vi "ziOpen.vi"(3 "Error In":errorcluster, 4 "Port obsolete (auto)":u16, 5 "Hostname obsolete (auto)":string, 6 "Address":string="DEV") -> (0 "Error Out":errorcluster, 1 "Selected Device":string, 2 "HandleOut":T1 {"Handle" format="0x%08x"; "Conn" format="0x%08x"})   [LabVIEW 2009, in "Zurich Instruments LabOne.lvlib"]
doc: "Creates a connection to a Data Server. <b>Address</b> is of the format {<host>}{:<port}{::<Device ID>}. Usually it is sufficient to provide the <b>Device ID</b> only. The host and port are then determined by network discovery. Should the discovery not work, prepend <host>:<port>:: to the Device ID. Examples are \"myhf2.company.com:8004::dev466\" or \"myhf2.company.com:8004\". In the latter case the first found instrument on the data server listening on myhf2.company.com:8004 will be selected."
uses:
  <instrlib>/Zurich Instruments LabOne/Zurich Instruments LabOne.lvlib
  <instrlib>/Zurich Instruments LabOne/Public/ziTypeHandle.ctl
  <instrlib>/Zurich Instruments LabOne/Public/ziTypeDisovery.ctl
  <instrlib>/Zurich Instruments LabOne/Private/ziLV64.dll
panel:
  out "auto-connected":bool
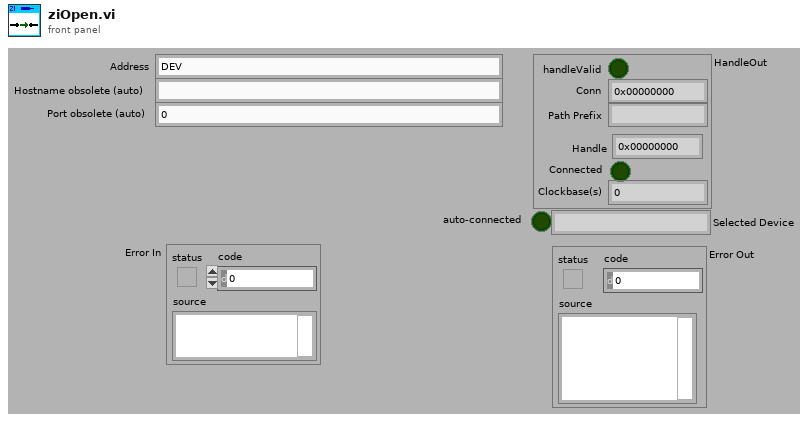
[diagram p1: front panel]
types:
  T1 = typedef "Zurich Instruments LabOne.lvlib/ziTypeHandle.ctl" = cluster{"handleValid":bool, "Conn":u64, "Path Prefix":string, "Handle":u64, "Connected":bool, "Clockbase(s)":dbl}
  T2 = typedef "Zurich Instruments LabOne.lvlib/ziTypeDisovery.ctl" = cluster{"timestamp":u64, "deviceid":string, "devicetype":string, "serveraddress":string, "serverport":u32, "apilevel":u32, "discoverable":bool, "interface":string, "connected":string, "available":bool, "owner":string, "status":string, "options ":string, "serverversion":string}
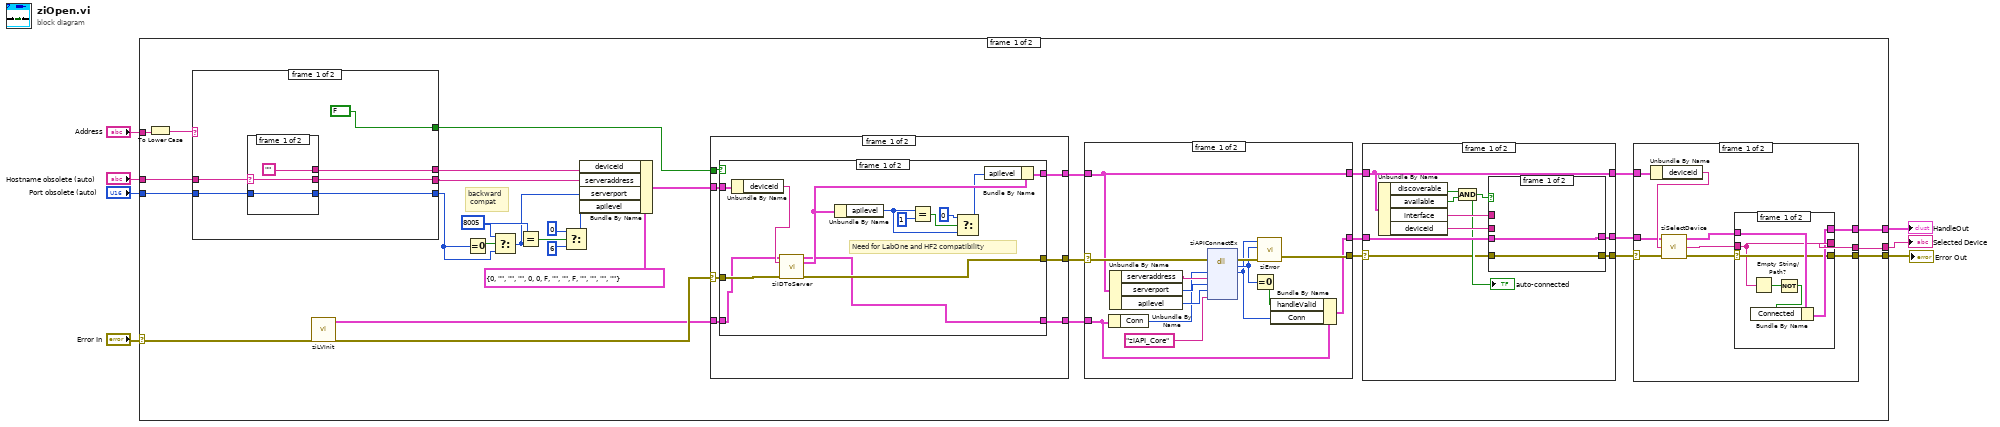
[diagram p0: block diagram]
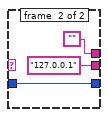
[diagram p2: hidden frame]
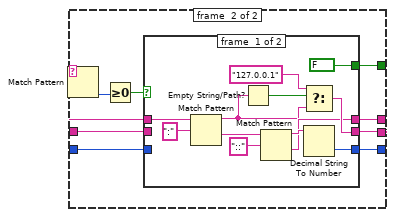
[diagram p3: hidden frame]
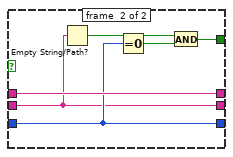
[diagram p4: hidden frame]
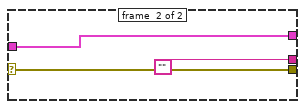
[diagram p6: hidden frame]
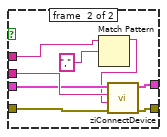
[diagram p7: hidden frame]
diagram:
  n1 = case shown="No Error" "Error In" {
    selector: "Error In" -> [w12 w168]
    tunnel: [w39 w168] -> w7
    tunnel: [w38 _] -> w6
    tunnel: "Hostname obsolete (auto)" -> [w31 _]
    tunnel: "Port obsolete (auto)" -> [w32 _]
    tunnel: [w37 _] -> w5
    tunnel: "Address" -> [w9 _]
    frame #0 {
      w18 = u32 8005
      # "backward\n compat"
      n2 = To Lower Case(string=w9) -> (all lower case string=w8:string)
      n3 = case shown="\"\", \"dev\"" w8 {
        selector: w8 -> [_ w54]
        tunnel: w31 -> [w45 w60]
        tunnel: w32 -> [w44 w56]
        tunnel: [w43 w61] -> w19
        tunnel: [w42 w59] -> w25
        tunnel: [w41 w58] -> w24
        tunnel: [FALSE w57] -> w21
        frame #0 {
          n4 = case shown="\"\"" w45 {
            selector: w45 -> [w47 _]
            tunnel: w44 -> [w46 w51]
            tunnel: [w46 w51] -> w43
            tunnel: [w47 "127.0.0.1"] -> w42
            tunnel: ["" ""] -> w41
            frame #0 {
            }
            frame #1 {
            }
          }
        }
        frame #1 {
          n5 = Match Pattern(string=w54, regular expression=":") -> (offset past match=w55:i32)  [unwired: 1 in, 3 out]
          n6 = Greater Or Equal To 0?(x=w55) -> (x >= 0?=w52:bool)
          n7 = case shown="False" w52 {
            tunnel: [w66 w78] -> w61
            tunnel: w60 -> [_ w75]
            tunnel: [w68 w75] -> w59
            tunnel: w54 -> [w72 w79]
            tunnel: [w65 w79] -> w58
            tunnel: [FALSE w76] -> w57
            tunnel: w56 -> [_ w78]
            frame #0 {
              n8 = Match Pattern(string=w72, regular expression=":") -> (before substring=w63:string, after substring=w69:string)  [unwired: 1 in, 2 out]
              n9 = Empty String/Path?(string/path=w63) -> (empty?=w62:bool)
              n10 = Match Pattern(string=w69, regular expression="::") -> (before substring=w67:string, after substring=w65:string)  [unwired: 1 in, 2 out]
              n11 = Select(t="127.0.0.1", s=w62, f=w63) -> (s? t:f=w68:string)
              n12 = Decimal String To Number(string=w67) -> (number=w66:i32)  [unwired: 2 in, 1 out]
            }
            frame #1 {
              n13 = Empty String/Path?(string/path=w75) -> (empty?=w74:bool)
              n14 = Equal To 0?(x=w78) -> (x = 0?=w77:bool)
              n15 = And(x=w74, y=w77) -> (x .and. y?=w76:bool)
            }
          }
        }
      }
      n16 = call <instrlib>:"ziLVInit.vi"("Error In"=w12) -> ("Error Out"=w11:errorcluster, "ziHandle"=w10:T1)  [unwired: 9 in]
      n17 = Equal To 0?(x=w19) -> (x = 0?=w20:bool)
      n18 = Select(t=w18, s=w20, f=w19) -> (s? t:f=w13:u32)
      n19 = Equal?(x=w18, y=w13) -> (x = y?=w17:bool)
      n20 = Select(t=u32 0, s=w17, f=u32 6) -> (s? t:f=w14:u32)
      n21 = Bundle By Name(cluster=T2 {"timestamp"=0, "deviceid"="", "devicetype"="", "serveraddress"="", "serverport"=0, "apilevel"=0, "discoverable"=FALSE, "interface"="", "connected"="", "available"=FALSE, "owner"="", "status"="", "options "="", "serverversion"=""} ("ziDiscovery"), "deviceid"=w24, "serveraddress"=w25, "serverport"=w13, "apilevel"=w14) -> (w27:T2)
      n22 = case shown="No Error" w11 {
        selector: w11 -> [w131 w150]
        tunnel: [w130 w150] -> w33
        tunnel: [w129 w148] -> w30
        tunnel: w21 -> [w128 _]
        tunnel: w27 -> [w127 w148]
        tunnel: w10 -> [w126 w149]
        tunnel: [w125 w149] -> w23
        frame #0 {
          n23 = case shown="True" w128 {
            tunnel: w131 -> [w144 w147]
            tunnel: [w143 w147] -> w130
            tunnel: [w141 w146] -> w129
            tunnel: w127 -> [w135 w146]
            tunnel: w126 -> [w132 w145]
            tunnel: [w133 w145] -> w125
            frame #0 {
              # "Need for LabOne and HF2 compatibility"
              n24 = Unbundle By Name(w135) -> ("deviceid"=w134:string)
              n25 = call <instrlib>:"ziIDToServer.vi"("ziHandle In"=w132, "Device ID"=w134, "Error In"=w144) -> ("ziHandle Out"=w133:T1, "ziDiscovery"=w142:T2, "Error Out"=w143:errorcluster)  [unwired: 10 in]
              n26 = Unbundle By Name(w142) -> ("apilevel"=w137:u32)
              n27 = Equal?(x=w137, y=u32 1) -> (x = y?=w139:bool)
              n28 = Select(t=u32 0, s=w139, f=w137) -> (s? t:f=w136:u32)
              n29 = Bundle By Name(cluster=w142, "apilevel"=w136) -> (w141:T2)
            }
            frame #1 {
            }
          }
        }
        frame #1 {
        }
      }
      n30 = case shown="No Error" w33 {
        selector: w33 -> [w160 w167]
        tunnel: [w163 w167] -> w34
        tunnel: w30 -> [w157 w166]
        tunnel: [w157 w166] -> w29
        tunnel: w23 -> [w153 w165]
        tunnel: [w152 w165] -> w22
        frame #0 {
          n31 = Unbundle By Name(w153) -> ("Conn"=w155:u64)
          n32 = Unbundle By Name(w157) -> ("serveraddress"=w159:string, "serverport"=w158:u32, "apilevel"=w156:u32)
          n33 = dll-call lib="C:/Program Files/National Instruments/LabVIEW 2009/instr.lib/Zurich Instruments LabOne/Private/ziLV*.*" fn="ziAPIConnectEx"(error in=w160, "Conn"=w155, "hostname"=w159, "Port"=w158, "ZIAPIVersion_enum"=w156, "Implementation"="ziAPI_Core") -> (error out=w164:errorcluster, "return type"=w162:u32, "Conn"=w154:u64)  [unwired: 6 in, 1 out]
          n34 = Equal To 0?(x=w162) -> (x = 0?=w151:bool)
          n35 = call <instrlib>:"ziError.vi"("Conn"=w154, "ziErrorCode"=w162, "Error In"=w164) -> ("Error Out"=w163:errorcluster)  [unwired: 3 in]
          n36 = Bundle By Name(cluster=w153, "handleValid"=w151, "Conn"=w154) -> (w152:T1)
        }
        frame #1 {
        }
      }
      n37 = case shown="No Error" w34 {
        selector: w34 -> [w102 w123]
        tunnel: w29 -> [w103 w122]
        tunnel: w22 -> [w110 w124]
        tunnel: [w109 w124] -> w36
        tunnel: [w108 w123] -> w35
        tunnel: [w103 w122] -> w28
        frame #0 {
          n38 = Unbundle By Name(w103) -> ("discoverable"=w105:bool, "available"=w106:bool, "interface"=w107:string, "deviceid"=w111:string)
          n39 = And(x=w105, y=w106) -> (x .and. y?=w104:bool)
          "auto-connected" <- w104
          n40 = case shown="True" w104 {
            tunnel: w111 -> [_ w121]
            tunnel: w110 -> [w112 w117]
            tunnel: [w112 w120] -> w109
            tunnel: [w113 w119] -> w108
            tunnel: w107 -> [_ w114]
            tunnel: w102 -> [w113 w118]
            frame #0 {
            }
            frame #1 {
              n41 = Match Pattern(string=w114, regular expression="," ("replace string (\"\")")) -> (before substring=w116:string)  [unwired: 1 in, 3 out]
              n42 = call <instrlib>:"ziConnectDevice.vi"("Error In"=w118, "Device Interface"=w116, "Device Serial"=w121, "Handle In"=w117) -> ("Error Out"=w119:errorcluster, "Handle Out"=w120:T1)  [unwired: 6 in]
            }
          }
        }
        frame #1 {
        }
      }
      n43 = case shown="No Error" w35 {
        selector: w35 -> [w89 w99]
        tunnel: [w80 w99] -> w39
        tunnel: w36 -> [w86 w101]
        tunnel: [w83 w101] -> w38
        tunnel: [w81 ""] -> w37
        tunnel: w28 -> [w88 _]
        frame #0 {
          n44 = Unbundle By Name(w88) -> ("deviceid"=w87:string)
          n45 = call <instrlib>:"ziSelectDevice.vi"("Error In"=w89, "Device (first)"=w87, "Handle In"=w86) -> ("Error Out"=w85:errorcluster, "Selected Device"=w82:string, "Handle Out"=w84:T1)
          n46 = case shown="No Error" w85 {
            selector: w85 -> [w93 w96]
            tunnel: w84 -> [w95 w98]
            tunnel: w82 -> [w92 w97]
            tunnel: [w94 w98] -> w83
            tunnel: [w92 w97] -> w81
            tunnel: [w93 w96] -> w80
            frame #0 {
              n47 = Empty String/Path?(string/path=w92) -> (empty?=w91:bool)
              n48 = Not(x=w91) -> (.not. x?=w90:bool)
              n49 = Bundle By Name(cluster=w95, "Connected"=w90) -> (w94:T1)
            }
            frame #1 {
            }
          }
        }
        frame #1 {
        }
      }
    }
    frame #1 {
    }
  }
  "Error Out" <- w7
  "HandleOut" <- w6
  "Selected Device" <- w5
